vi "LS4 ConnectSimpleSD.vi"(1 "Show Protocol":bool=TRUE, 3 "I/O Adress (DPRAM)":u32=832 format="%.0x", 4 "Baudrate":u16=9600, 5 "COM Port":u32=1, 6 "Interface (1: RS232; 2: ArcNet; 3: DPRAM)":u32=1) -> (0 "Initialization OK":bool=TRUE)   [LabVIEW 2015]
doc: "This VI opens a connection to the LStep control. \n\nInterface selects the interface type:\n1 = RS232\n2 = ArcNet\n3 = ISA/DPRAM\n\nset ComPort = 1 to select 'COM1'\n\nBaudRate = 9600 or 57600 (RS232)\n\nI/O Adress is the base adress of the LSTEP-PC card (only DPRAM)"
uses:
  DLL/LStep4.dll
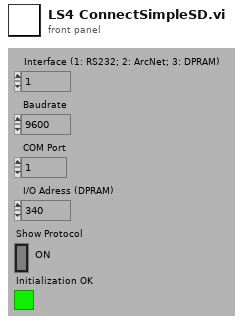
[diagram p1: front panel]
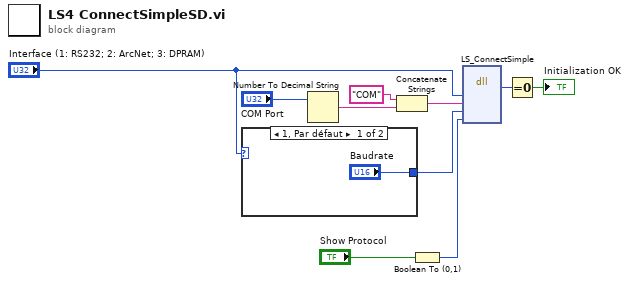
[diagram p0: block diagram]
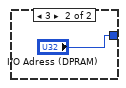
[diagram p2: hidden frame]
diagram:
  n1 = case shown="1, Par défaut" "Interface (1: RS232; 2: ArcNet; 3: DPRAM)" {
    tunnel: ["Baudrate" "I/O Adress (DPRAM)"] -> w5
    frame 1, Default {
    }
    frame 3 {
    }
  }
  n2 = Number To Decimal String(number="COM Port") -> (decimal integer string=w7:string)  [unwired: 1 in]
  n3 = Concatenate Strings("COM", w7) -> (w9:string)
  n4 = Boolean To (0,1)(Boolean="Show Protocol") -> (0, 1=w2:i16)
  n5 = dll-call lib="G:/SD/TRANCON/DLL/LStep4.dll" fn="LS_ConnectSimple" ("Call Library Function")("AnInterfaceType"="Interface (1: RS232; 2: ArcNet; 3: DPRAM)", "AComName"=w9, "ABR"=w5, "AShowProt"=w2) -> ("type de retour"=w1:i32)  [unwired: 7 in, 2 out]
  n6 = Equal To 0?(x=w1) -> (x = 0?=→"Initialization OK":bool)
